vi "Execute.vi"(8 "error in (no error)":errorcluster caption="Fehler (Eingang, kein Fehler)", 9 "WhereIGetMyInformation":string, 10 "WhoIAm":string, 11 "ApllicationLoadAndConfigurationClass Eingang":refnum<class "LoadConfigurationClass.lvclass"> caption="DNL_LabVIEW Object in") -> (0 "error out":errorcluster caption="Fehler (Ausgang)", 2 "DictionaryString.lvclass":refnum<class "DictionaryString.lvclass">, 3 "ApllicationLoadAndConfigurationClass Ausgang":refnum<class "LoadConfigurationClass.lvclass"> caption="DNL_LabVIEW Object out")   [LabVIEW 2013, in "LoadConfigurationClass.lvclass"]
uses:
  LoadConfigurationClass.lvclass
  DictionaryStringClass/DictionaryString.lvclass
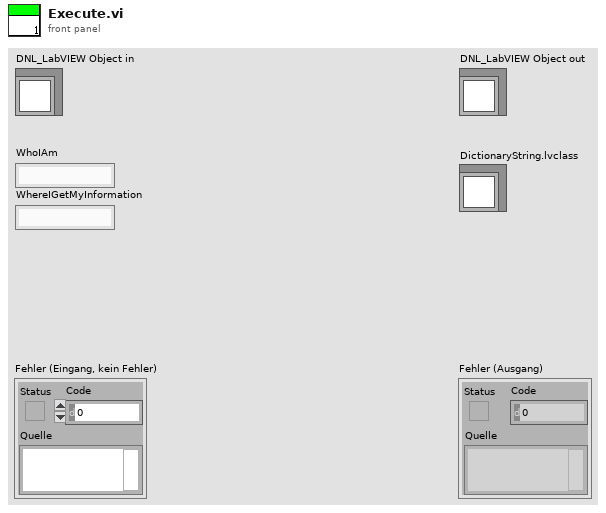
[diagram p1: front panel]
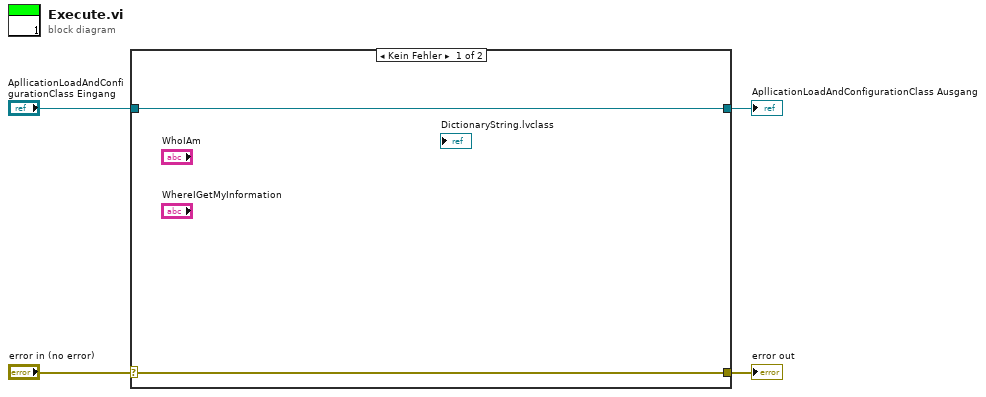
[diagram p0: block diagram]
diagram:
  n1 = case shown="Kein Fehler" "error in (no error)" {
    selector: "error in (no error)" -> [w6 w8]
    tunnel: [w6 w8] -> w3
    tunnel: [w5 w7] -> w1
    tunnel: "ApllicationLoadAndConfigurationClass Eingang" -> [w5 w7]
    frame No Error {
    }
    frame Error {
    }
  }
  "error out" <- w3
  "ApllicationLoadAndConfigurationClass Ausgang" <- w1
